vi "EstimateGamepiece.vi"(0 "Odometry Timestamp (ms)":u32, 5 "X (in) [t0]":dbl, 7 "Y (in) [t0]":dbl, 9 "Confidence":dbl, 11 "Vision Timestamp (ms)":u32, 12 "Gamepiece X":dbl, 13 "Gamepiece Y":dbl, 14 "piece?":enum16{"Cube", "Cone", "None"}(ring)) -> (8 "Seen_Game_Pieces":T1(array[cluster]))   [LabVIEW 2020]
uses:
  628b9fa5-cf97-4d01-a47b-77a292797d37.vi
  dbd7e9ae-d3d7-4685-be97-b0d109e1f5b7.vi
  b7d6566a-2419-425d-af50-6320a3cd7c5b.vi
  8b8e666f-6eb4-4d19-ae86-86583ba98964.vi
  a3d5a9e1-9ff1-4e55-8265-c989f82d1d85.vi
  b9bae949-81c7-4c67-942b-ceedbbe4297c.vi
  GlobalPoseAndTargeting.vi
  GlobalArm.vi
  <vilib>/Comparison/Equal/Equal Functor/Equal Functor.lvclass
panel:
  out "size(s)":i32
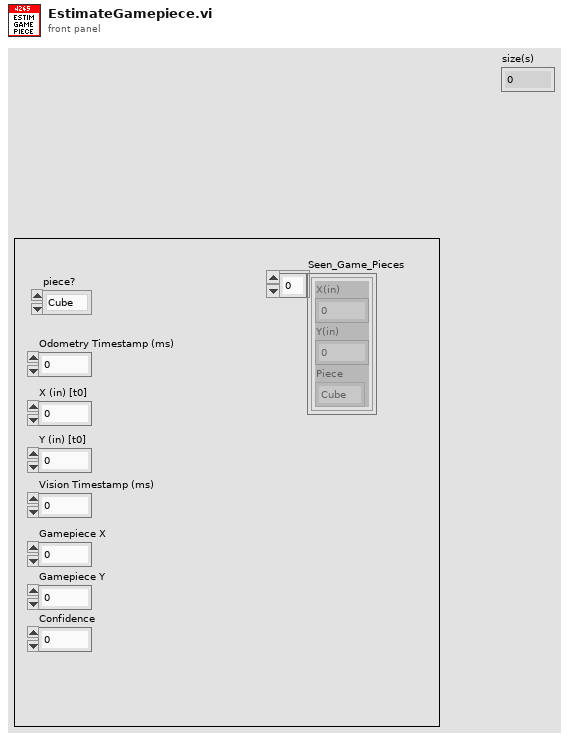
[diagram p1: front panel]
types:
  T1 = cluster{"X(in)":dbl, "Y(in)":dbl, "Piece":enum16{"Cube", "Cone"}}[]
  T2 = cluster{"X":dbl, "Y":dbl, "Vision Timestamp (ms)":u32, "Confidence":dbl, "Range":dbl, "piece? 2":enum16{"Cube", "Cone", "None"}}[]
  T3 = cluster{"X":dbl, "Y":dbl, "Vision Timestamp (ms)":u32, "Confidence":dbl, "Range":dbl, "Piece":enum16{"Cube", "Cone"}}[][]
  T4 = cluster{"X":dbl, "Y":dbl, "Vision Timestamp (ms)":u32, "Confidence":dbl, "Range":dbl, "piece? 2":enum16{"Cube", "Cone", "None"}}
  T5 = cluster{"X":dbl, "Y":dbl, "Vision Timestamp (ms)":u32, "Confidence":dbl, "Range":dbl, "Piece":enum16{"Cube", "Cone"}}[]
  T6 = cluster{"X(in)":dbl, "Y(in)":dbl, "Count":i32, "Timestamp(ms)":u32, "Piece":enum16{"Cube", "Cone"}}
  T7 = cluster{"X":dbl, "Y":dbl, "Vision Timestamp (ms)":u32, "Confidence":dbl, "Range":dbl, "Piece":enum16{"Cube", "Cone"}}
  T8 = cluster{"X(in)":dbl, "Y(in)":dbl, "Piece":enum16{"Cube", "Cone"}}
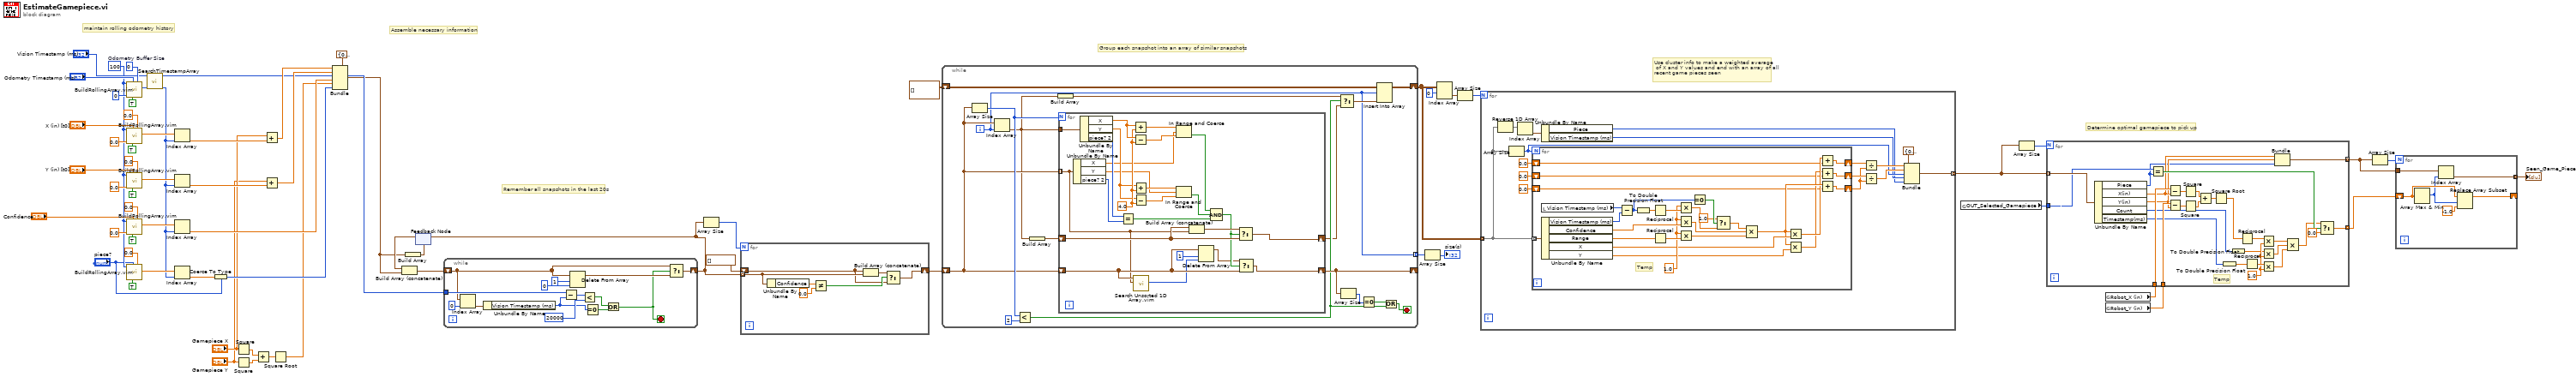
[diagram p0: block diagram]
diagram:
  w18 = 100  # Odometry Buffer Size
  # "Determine optimal gamepiece to pick up"
  # "Use cluster info to make a weighted average\n of X and Y values and end with an array of all recent game pieces seen"
  # "Group each snapshot into an array of similar snapshots"
  # "Remember all snapshots in the last 20s"
  # "Assemble necessary information"
  # "maintain rolling odometry history"
  n1 = call "BuildRollingArray.vim"("Global Additive Update"=0, "Update?"=TRUE, "New Value"="Odometry Timestamp (ms)", "Initial Value"=0, "Number of Elements"=w18) -> ("Current Array"=w61:u32[])  [unwired: 6 in]
  n2 = call "BuildRollingArray.vim"("Global Additive Update"=0.0, "Update?"=TRUE, "New Value"="X (in) [t0]", "Initial Value"=0.0, "Number of Elements"=w18) -> ("Current Array"=w60:dbl[])  [unwired: 6 in]
  n3 = call "BuildRollingArray.vim"("Global Additive Update"=0.0, "Update?"=TRUE, "New Value"="Y (in) [t0]", "Initial Value"=0.0, "Number of Elements"=w18) -> ("Current Array"=w59:dbl[])  [unwired: 6 in]
  n4 = call "BuildRollingArray.vim"("Global Additive Update"=0.0, "Update?"=TRUE, "New Value"="Confidence", "Initial Value"=0.0, "Number of Elements"=w18) -> ("Current Array"=w41:dbl[])  [unwired: 6 in]
  n5 = call "BuildRollingArray.vim"("Global Additive Update"=0.0, "Update?"=TRUE, "New Value"="piece?", "Number of Elements"=w18) -> ("Current Array"=w33:dbl[])  [unwired: 7 in]
  n6 = call "SearchTimestampArray.vi"("Timestamp Array"=w61, "Search Timestamp"="Vision Timestamp (ms)") -> ("Closest Index"=w17:i32)  [unwired: 8 in, 1 out]
  n7 = Index Array(array=w60, index=w17) -> (element=w24:dbl)
  n8 = Index Array(array=w59, index=w17) -> (element=w25:dbl)
  n9 = Index Array(array=w41, index=w17) -> (element=w37:dbl)
  n10 = Index Array(array=w33, index=w17) -> (element=w32:dbl)
  n11 = Coerce To Type(0:w32, 1:"piece?") -> (2:w31:enum16{"Cube", "Cone", "None"})
  n12 = Square(x="Gamepiece X") -> (x^2=w47:dbl)
  n13 = Square(x="Gamepiece Y") -> (x^2=w46:dbl)
  n14 = Add(x=w47, y=w46) -> (x+y=w48:dbl)
  n15 = Add(x="Gamepiece X", y=w24) -> (x+y=w50:dbl)
  n16 = Add(x="Gamepiece Y", y=w25) -> (x+y=w49:dbl)
  n17 = Square Root(x=w48) -> (sqrt(x)=w16:dbl)
  n18 = Bundle(cluster=T4 {"X"=0.0, "Y"=0.0, "Vision Timestamp (ms)"=0, "Confidence"=0.0, "Range"=0.0, "piece? 2"=enum."Cube"} ("Cluster"), "X"=w50, "Y"=w49, "Vision Timestamp (ms)"="Vision Timestamp (ms)", "Confidence"=w37, "Range"=w16, "piece? 2"=w31) -> (w8:T4)
  n19 = Build Array(w8) -> (w7:T2)
  n20 = feedback #1(w7) -> (w23:T2)
  n21 = Build Array (concatenate)(w23, w8) -> (w9:T2)
  n22 = while {
    tunnel: "Vision Timestamp (ms)" -> [w77]
    shift-right: [w70] -> w5
    shift-left: w9 -> [w72]
    stop <- w66 stop-if-true
    n23 = Index Array(array=w72, index=0) -> (element=w78:T4)
    n24 = Unbundle By Name(w78) -> ("Vision Timestamp (ms)"=w69:u32)
    n25 = Subtract(x=w77, y=w69) -> (x-y=w76:u32)
    n26 = Delete From Array(array=w72, length=1, index=0) -> (array with subset deleted=w71:T2)  [unwired: 1 out]
    n27 = Less?(x=w76, y=u32 20000) -> (x < y?=w67:bool)
    n28 = Equal To 0?(x=w69) -> (x = 0?=w68:bool)
    n29 = Or(x=w67, y=w68) -> (x .or. y?=w66:bool)
    n30 = Select(t=w72, s=w66, f=w71) -> (s? t:f=w70:T2)
  }
  n31 = feedback-in #1(w5) -> ()
  n32 = Array Size(array=w5) -> (size(s)=w6:i32)
  n33 = for {
    N: w6 -> [_]
    tunnel: w5 -> [w83] mode=indexing
    shift-right: [w82] -> w4
    shift-left: T2 [] -> [w81]
    n34 = Unbundle By Name(w83) -> ("Confidence"=w86:dbl)
    n35 = Not Equal?(x=w86, y=0.0) -> (x != y?=w84:bool)
    n36 = Build Array (concatenate)(w81, w83) -> (w85:T2)
    n37 = Select(t=w85, s=w84, f=w81) -> (s? t:f=w82:T2)
  }
  n38 = while {
    shift-right: [w101] -> _
    shift-left: w4 -> [w94]
    shift-right: [w92] -> w13
    shift-left: T3 [] -> [w91]
    tunnel: [w87] -> w3 mode=indexing
    i -> [w87]
    stop <- w96 stop-if-true
    n39 = Array Size(array=w94) -> (size(s)=w99:i32)
    n40 = Index Array(array=w94, index=w87) -> (element=w93:T4)
    n41 = Less?(x=w99, y=2) -> (x < y?=w95:bool)
    n42 = Build Array(w93) -> (w102:T2)
    n43 = Build Array(w93) -> (w89:T2)
    n44 = for {
      N: w99 -> [_]
      tunnel: w93 -> [w113]
      shift-right: [w110] -> w88
      shift-left: w102 -> [w112]
      tunnel: w94 -> [w104] mode=indexing
      shift-right: [w109] -> w101
      shift-left: w94 -> [w105]
      w122 = 4.0
      n45 = Unbundle By Name(w104) -> ("X"=w114:dbl, "Y"=w115:dbl, "piece? 2"=w116:enum16{"Cube", "Cone", "None"})
      n46 = Unbundle By Name(w113) -> ("X"=w126:dbl, "Y"=w121:dbl, "piece? 2"=w120:enum16{"Cube", "Cone", "None"})
      n47 = Equal?(x=w120, y=w116) -> (x = y?=w117:bool)
      n48 = Add(x=w126, y=w122) -> (x+y=w127:dbl)
      n49 = Subtract(x=w126, y=w122) -> (x-y=w125:dbl)
      n50 = Add(x=w121, y=w122) -> (x+y=w124:dbl)
      n51 = Subtract(x=w121, y=w122) -> (x-y=w123:dbl)
      n52 = call "Search Unsorted 1D Array.vim"("element"=w104, "unsorted 1D array"=w105) -> ("index of element"=w103:i32)  [unwired: 9 in]
      n53 = In Range and Coerce(upper limit=w127, x=w114, lower limit=w125) -> (In Range?=w119:bool)  [unwired: 1 out]
      n54 = In Range and Coerce(upper limit=w124, x=w115, lower limit=w123) -> (In Range?=w118:bool)  [unwired: 1 out]
      n55 = Build Array (concatenate)(w112, w104) -> (w111:T2)
      n56 = Delete From Array(array=w105, length=1, index=w103) -> (array with subset deleted=w106:T2)  [unwired: 1 out]
      n57 = Compound Arithmetic op=AND(w119, w118, w117) -> (w108:bool)
      n58 = Select(t=w111, s=w108, f=w112) -> (s? t:f=w110:T2)
      n59 = Select(t=w106, s=w108, f=w105) -> (s? t:f=w109:T2)
    }
    n60 = Select(t=w89, s=w95, f=w88) -> (s? t:f=w90:T2)
    n61 = Array Size(array=w101) -> (size(s)=w100:i32)
    n62 = Equal To 0?(x=w100) -> (x = 0?=w97:bool)
    n63 = Insert Into Array(array=w91, index (row)=w87, new element=w90) -> (w92:T3)  [unwired: 1 in]
    n64 = Or(x=w97, y=w95) -> (x .or. y?=w96:bool)
  }
  n65 = Array Size(array=w3) -> (size(s)=→"size(s)":i32)
  n66 = Index Array(array=w13, index (row)=0) -> (element=w43:T5)  [unwired: 1 in]
  n67 = Array Size(array=w43) -> (size(s)=w44:i32)
  n68 = for {
    N: w44 -> [_]
    tunnel: w13 -> [w132] mode=indexing
    tunnel: [w128] -> w26 mode=indexing
    n69 = Reverse 1D Array(array=w132) -> (reversed array=w131:T5)
    n70 = Array Size(array=w132) -> (size(s)=w135:i32)
    n71 = Index Array(array=w131) -> (element=w134:T7)  [unwired: 1 in]
    n72 = for {
      N: w135 -> [_]
      tunnel: w132 -> [w149] mode=indexing
      shift-right: [w154] -> w140
      shift-left: 0.0 -> [w155]
      shift-right: [w152] -> w139
      shift-left: 0.0 -> [w153]
      shift-right: [w150] -> w138
      shift-left: 0.0 -> [w151]
      w162 = 1.0 ("x")
      # "Temp"
      n73 = Unbundle By Name(w149) -> ("Vision Timestamp (ms)"=w170:u32, "Confidence"=w165:dbl, "Range"=w168:dbl, "X"=w160:dbl, "Y"=w158:dbl)
      n74 = local read "Vision Timestamp (ms)"() -> (w169:u32)
      n75 = Subtract(x=w169, y=w170) -> (x-y=w147:u32)
      n76 = To Double Precision Float(number=w147) -> (double precision float=w167:dbl)
      n77 = Reciprocal(x=w167) -> (1/x=w166:dbl)
      n78 = Reciprocal(x=w168) -> (1/x=w163:dbl)
      n79 = Multiply(x=w162, y=w166) -> (x*y=w144:dbl)
      n80 = Multiply(x=w162, y=w165) -> (x*y=w164:dbl)
      n81 = Multiply(x=w162, y=w163) -> (x*y=w161:dbl)
      n82 = Equal To 0?(x=w147) -> (x = 0?=w146:bool)
      n83 = Select(t=1.0, s=w146, f=w144) -> (s? t:f=w148:dbl)
      n84 = Compound Arithmetic op=MULTIPLY(w148, w164, w161) -> (w159:dbl)
      n85 = Multiply(x=w159, y=w160) -> (x*y=w157:dbl)
      n86 = Multiply(x=w159, y=w158) -> (x*y=w156:dbl)
      n87 = Add(x=w157, y=w155) -> (x+y=w154:dbl)
      n88 = Add(x=w156, y=w153) -> (x+y=w152:dbl)
      n89 = Add(x=w159, y=w151) -> (x+y=w150:dbl)
    }
    n90 = Unbundle By Name(w134) -> ("Piece"=w130:enum16{"Cube", "Cone"}, "Vision Timestamp (ms)"=w133:u32)
    n91 = Divide(x=w140, y=w138) -> (x/y=w137:dbl)
    n92 = Divide(x=w139, y=w138) -> (x/y=w136:dbl)
    n93 = Bundle(cluster=T6 {"X(in)"=0.0, "Y(in)"=0.0, "Count"=0, "Timestamp(ms)"=0, "Piece"=enum."Cube"}, "X(in)"=w137, "Y(in)"=w136, "Count"=w135, "Timestamp(ms)"=w133, "Piece"=w130) -> (w128:T6)
  }
  n94 = global read "GlobalArm.vi" "OUT_Selected_Gamepiece"() -> (w27:enum16{"Cube", "Cone"})
  n95 = Array Size(array=w26) -> (size(s)=w36:i32)
  n96 = global read "GlobalPoseAndTargeting.vi" "Robot_X (in)"() -> (w29:dbl)
  n97 = global read "GlobalPoseAndTargeting.vi" "Robot_Y (in)"() -> (w28:dbl)
  n98 = for {
    N: w36 -> [_]
    tunnel: w26 -> [w198] mode=indexing
    tunnel: w29 -> [w197]
    tunnel: w28 -> [w196]
    tunnel: w27 -> [w178]
    tunnel: [w175] -> w21 mode=indexing
    tunnel: [w171] -> w20 mode=indexing
    w183 = 1.0
    # "Temp"
    n99 = Unbundle By Name(w198) -> ("Piece"=w172:enum16{"Cube", "Cone"}, "X(in)"=w174:dbl, "Y(in)"=w173:dbl, "Count"=w188:i32, "Timestamp(ms)"=w187:u32)
    n100 = Equal?(x=w178, y=w172) -> (x = y?=w190:bool)
    n101 = Subtract(x=w197, y=w174) -> (x-y=w195:dbl)
    n102 = Subtract(x=w196, y=w173) -> (x-y=w194:dbl)
    n103 = Square(x=w195) -> (x^2=w193:dbl)
    n104 = Square(x=w194) -> (x^2=w192:dbl)
    n105 = Add(x=w193, y=w192) -> (x+y=w191:dbl)
    n106 = Square Root(x=w191) -> (sqrt(x)=w189:dbl)
    n107 = To Double Precision Float(number=w187) -> (double precision float=w184:dbl)
    n108 = To Double Precision Float(number=w188) -> (double precision float=w182:dbl)
    n109 = Reciprocal(x=w189) -> (1/x=w185:dbl)
    n110 = Reciprocal(x=w184) -> (1/x=w186:dbl)
    n111 = Multiply(x=w185, y=w183) -> (x*y=w181:dbl)
    n112 = Multiply(x=w182, y=w183) -> (x*y=w180:dbl)
    n113 = Multiply(x=w186, y=w183) -> (x*y=w179:dbl)
    n114 = Bundle("X(in)"=w174, "Y(in)"=w173, "Piece"=w172) -> (w171:T8)  [unwired: 1 in]
    n115 = Compound Arithmetic op=MULTIPLY(w181, w180, w179) -> (w177:dbl)
    n116 = Select(t=w177, s=w190, f=0.0) -> (s? t:f=w175:dbl)
  }
  n117 = Array Size(array=w20) -> (size(s)=w22:i32)
  n118 = for {
    N: w22 -> [_]
    tunnel: w20 -> [w204]
    shift-right: [w202] -> _
    shift-left: w21 -> [w201]
    tunnel: [w203] -> w19 mode=indexing
    n119 = Array Max & Min(array=w201) -> (max index (indices)=w199:i32)  [unwired: 3 out]
    n120 = Index Array(array=w204, index=w199) -> (element=w203:T8)
    n121 = Replace Array Subset(array=w201, new element=-1.0 ("new element/subarray"), index=w199) -> (w202:dbl[])
  }
  "Seen_Game_Pieces" <- w19
